vi "Day 7.1 - align crabs subs.vi"(11 "input":i32[](array[numeric])) -> (3 "output":i32)   [LabVIEW 2021]
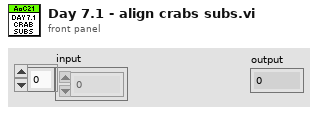
[diagram p1: front panel]
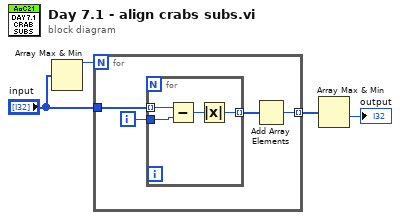
[diagram p0: block diagram]
diagram:
  n1 = Array Max & Min(array="input") -> (max value=w3:i32)  [unwired: 3 out]
  n2 = for {
    N: w3 -> [_]
    tunnel: "input" -> [w8]
    tunnel: [w6] -> w2 mode=indexing
    i -> [w5]
    n3 = for {
      tunnel: w5 -> [w11]
      tunnel: w8 -> [w12] mode=indexing
      tunnel: [w9] -> w7 mode=indexing
      n4 = Subtract(x=w12, y=w11) -> (x-y=w10:i32)
      n5 = Absolute Value(x=w10) -> (abs(x)=w9:i32)
    }
    n6 = Add Array Elements(numeric array=w7) -> (sum=w6:i32)
  }
  n7 = Array Max & Min(array=w2) -> (min value=→"output":i32)  [unwired: 3 out]
